vi "Read CSM API with lvcsm Support.vi"(6 "Config Path(\"\" for lvcsm file)":path, 7 "Current Module(\"\" to generate a ID)":string, 8 "error in (no error)":errorcluster, 9 "Force?(F)":bool, 11 "CSM Name":string) -> (0 "Error out":errorcluster, 3 "CSMAPI List":string[](array[string]))   [LabVIEW 2017, in "CSM-Helper API with lvcsm Support.lvlib"]
uses:
  CSM-Helper API with lvcsm Support.lvlib
  Properties/Read APIs.vi
  CSM-Helper.lvclass
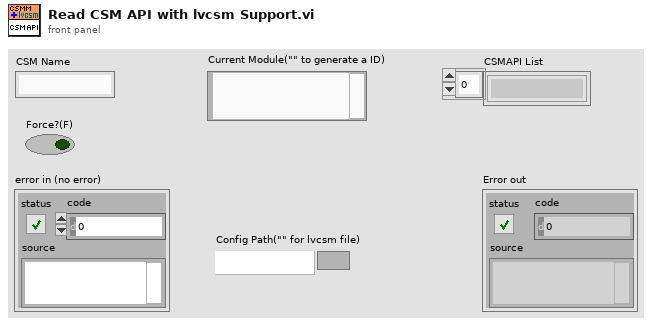
[diagram p1: front panel]
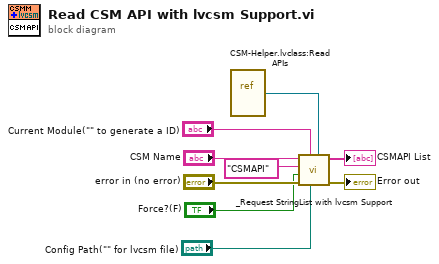
[diagram p0: block diagram]
diagram:
  n1 = vi-ref "CSM-Helper.lvclass:Read APIs.vi"() -> (w2:refnum<vi>)
  n2 = call "_Request StringList with lvcsm Support.vi"("API Ref"=w2, "Config Path(\"\" for lvcsm file)"="Config Path(\"\" for lvcsm file)", "Current Module(\"\" to generate a ID)"="Current Module(\"\" to generate a ID)", "error in (no error)"="error in (no error)", "Force?(F)"="Force?(F)", "API Name"="CSMAPI", "CSM Name"="CSM Name") -> ("Error out"=→"Error out":errorcluster, "CSMAPI List"=→"CSMAPI List":string[])  [unwired: 3 in]
